vi "4_3.vi"() -> ()   [LabVIEW 2018]
panel:
  in  "stop (T)":bool=TRUE
  out "Waveform Graph":dynamicdata(graph)
  out "Numeric":dbl
  in  "stop":bool
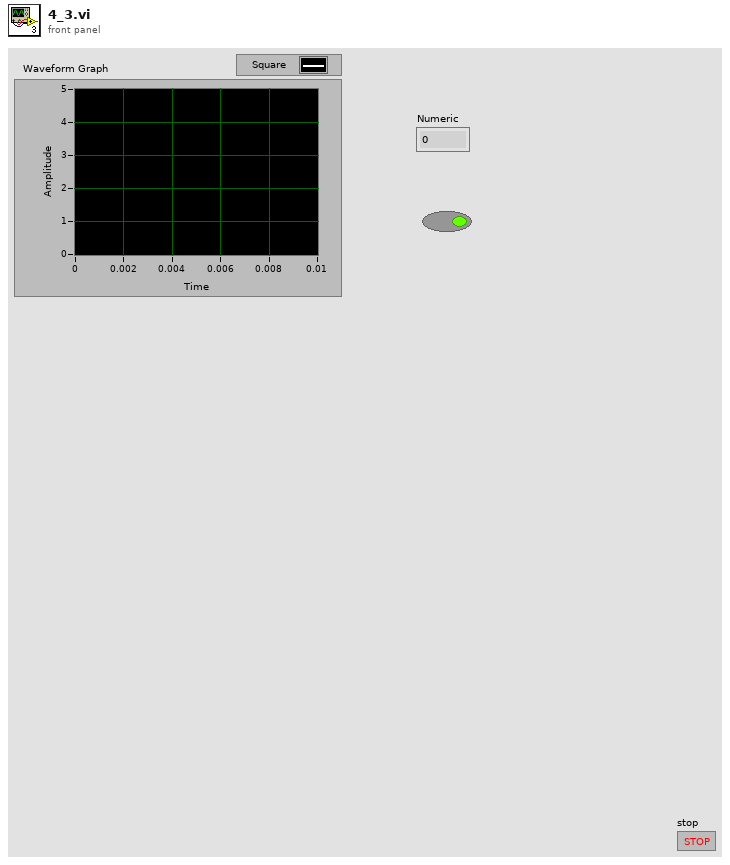
[diagram p1: front panel]
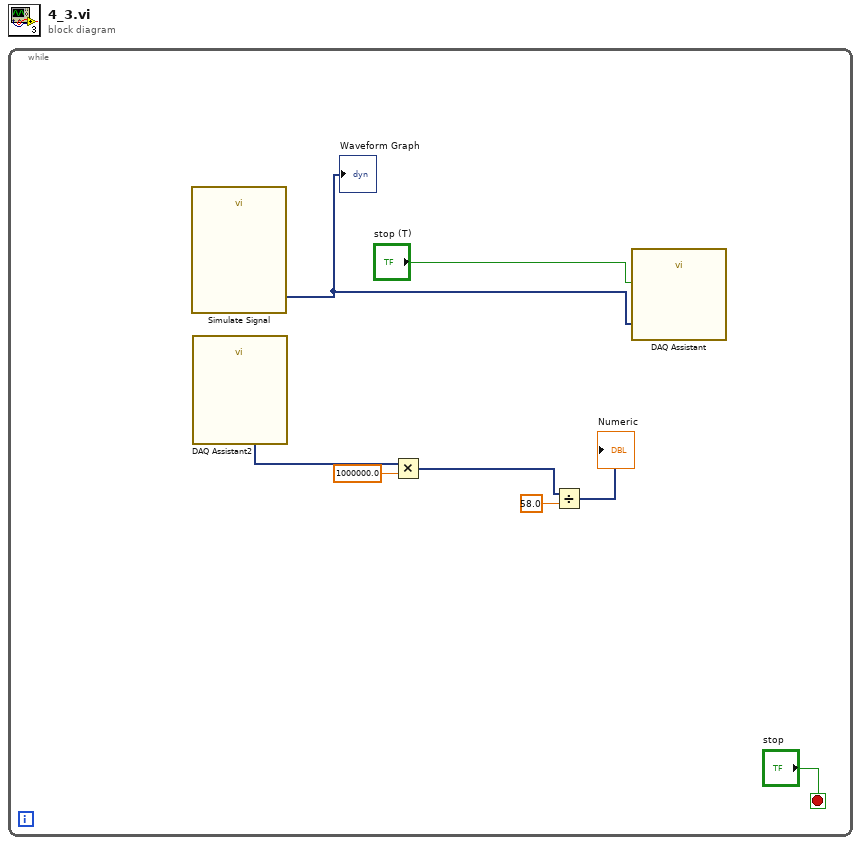
[diagram p0: block diagram]
diagram:
  n1 = while {
    stop <- "stop" stop-if-true
    n2 = call "Simulate Signal"() -> ("Square"=w3:dynamicdata)  [unwired: 14 in, 1 out]
    "Waveform Graph" <- w3
    n3 = call "DAQ Assistant2"() -> ("data"=w7:dynamicdata)  [unwired: 16 in, 3 out]
    n4 = Multiply(x=w7, y=1000000.0) -> (x*y=w5:dynamicdata)
    n5 = Divide(x=w5, y=58.0) -> (x/y=→"Numeric":dynamicdata)
    n6 = call "DAQ Assistant"("data"=w3, "stop (F)"="stop (T)") -> ()  [unwired: 15 in, 3 out]
  }
